vi "Create Text Form.vi"(6 "Color":u32(colorbox), 7 "[user-specified font]":T1, 8 "error in (no error)":errorcluster, 9 "Origin":cluster{"horizontal":i16, "vertical":i16}, 10 "Text":string, 11 "Text in":refnum<class "Text.lvclass">) -> (0 "error out":errorcluster, 3 "New Text":refnum<class "Text.lvclass">)   [LabVIEW 2015, in "LV Image Editor Framework.lvlib" / "Text.lvclass"]
uses:
  Text.lvclass
  Text.lvclass/Text.ctl
  Shape/Shape.lvclass/Shape.ctl
  Shape/Write Color.vi
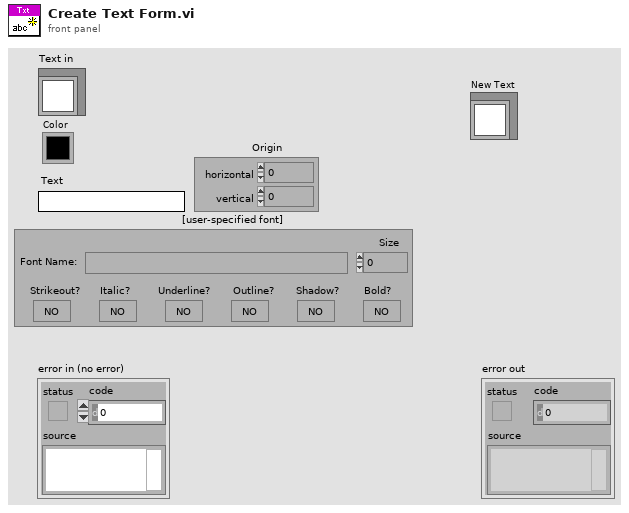
[diagram p1: front panel]
types:
  T1 = cluster{"Font Name:":string, "Size":i16, "Strikeout?":bool, "Italic?":bool, "Underline?":bool, "Outline?":bool, "Shadow?":bool, "Bold?":bool}
  T2 = enum16{"User-specified Font", "Application Font", "System Font", "Dialog Font"}
  T3 = cluster{"left":i16, "top":i16, "right":i16, "bottom":i16}
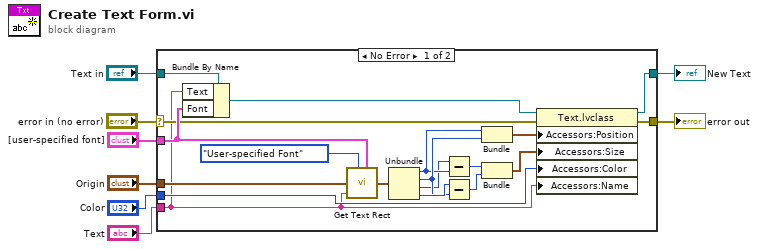
[diagram p0: block diagram]
diagram:
  n1 = case shown="No Error" "error in (no error)" {
    selector: "error in (no error)" -> [w11 w29]
    tunnel: [w12 w29] -> w7
    tunnel: [w13 w28] -> w1
    tunnel: "Text in" -> [w17 w28]
    tunnel: "Text" -> [w9 _]
    tunnel: "[user-specified font]" -> [w19 _]
    tunnel: "Origin" -> [w27 _]
    tunnel: "Color" -> [w14 _]
    frame No Error {
      n2 = Bundle By Name(cluster=w17, "Text"=w9, "Font"=w19) -> (w16:refnum<class "Text.lvclass">)
      n3 = call <vilib>:"Get Text Rect.vi"("desired font(Application)"=T2."User-specified Font", "origin(0,0)"=w27, "text"=w9, "[user-specified font]"=w19) -> ("rect"=w26:T3)  [unwired: 5 in]
      n4 = Unbundle(w26) -> ("left"=w23:i16, "top"=w24:i16, "right"=w22:i16, "bottom"=w25:i16)
      n5 = Subtract(x=w22, y=w23) -> (x-y=w21:i16)
      n6 = Subtract(x=w25, y=w24) -> (x-y=w20:i16)
      n7 = Bundle("left"=w23, "top"=w24) -> (w10:cluster{"left":i16, "top":i16})  [unwired: 1 in]
      n8 = Bundle(w21, w20) -> (w15:cluster{i16, i16})  [unwired: 1 in]
      n9 = property class="Text.lvclass"(reference=w16, error in=w11, "Accessors:Position"=w10, "Accessors:Size"=w15, "Accessors:Color"=w14, "Accessors:Name"=w9) -> (reference out=w13:refnum<class "Text.lvclass">, error out=w12:errorcluster)
    }
    frame Error {
    }
  }
  "error out" <- w7
  "New Text" <- w1
